vi "Write Incoming Work Dispatcher.vi"(8 "error in (no error)":errorcluster, 10 "Incoming Work Dispatcher Queue":refnum<class "Message Enqueuer.lvclass">, 11 "Worker in":refnum<class "Worker.lvclass">) -> (0 "error out":errorcluster, 3 "Worker out":refnum<class "Worker.lvclass">)   [LabVIEW 2023, in "Worker.lvlib" / "Worker.lvclass"]
doc: "Simple accessor method to set the <b>Incoming Work Dispatcher</b> enqueuer reference of the <b>Worker</b>. \n\nThe Incoming Work Dispatcher is the Actor responsible for giving the Worker tasks to complete. The enqueuer reference is used by the Worker to signal that it is available for a new task."
uses:
  Worker.lvclass
  <vilib>/ActorFramework/Message Enqueuer/Message Enqueuer.lvclass
  Worker.lvclass/Worker.ctl
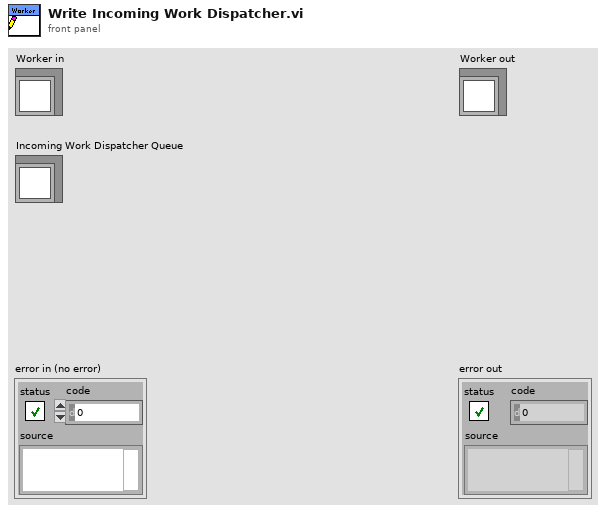
[diagram p1: front panel]
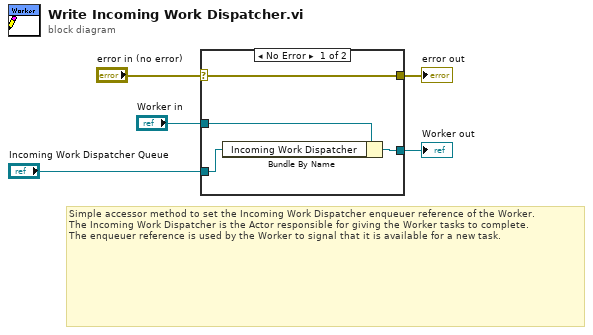
[diagram p0: block diagram]
diagram:
  # "Simple accessor method to set the Incoming Work Dispatcher enqueuer reference of the Worker.  \nThe Incoming Work Dispatcher is the Actor responsible for giving the Worker tasks to complete.  \nThe enqueuer reference is used by the Worker to signal that it is available for a new task."
  n1 = case shown="No Error" "error in (no error)" {
    selector: "error in (no error)" -> [w9 w10]
    tunnel: [w9 w10] -> w4
    tunnel: [w7 w11] -> w2
    tunnel: "Worker in" -> [w8 w11]
    tunnel: "Incoming Work Dispatcher Queue" -> [w6 _]
    frame No Error {
      n2 = Bundle By Name(cluster=w8, "Incoming Work Dispatcher"=w6) -> (w7:refnum<class "Worker.lvclass">)
    }
    frame Error {
    }
  }
  "error out" <- w4
  "Worker out" <- w2
